vi "SSC DCPower Source Current v2.vi"(0 "DCPower SSC in":T1[](array[typedef]), 5 "Voltage Limit, V":dbl, 9 "Voltage Limit Range (V)":dbl format="%#_6p", 11 "error in":errorcluster, 12 "Current Level Range (A)":dbl=0.001 format="%#_13p", 14 "Current Level (A)":dbl format="%#_13g") -> (4 "DCPower SSC out":T1[](array[typedef]), 15 "error out":errorcluster)   [LabVIEW 2019]
uses:
  SSC DCPower.ctl
  <instrlib>/niDCPower/nidcpower.llb/niDCPower Output Function.ctl
  <instrlib>/niDCPower/nidcpower.llb/niDCPower Source Mode.ctl
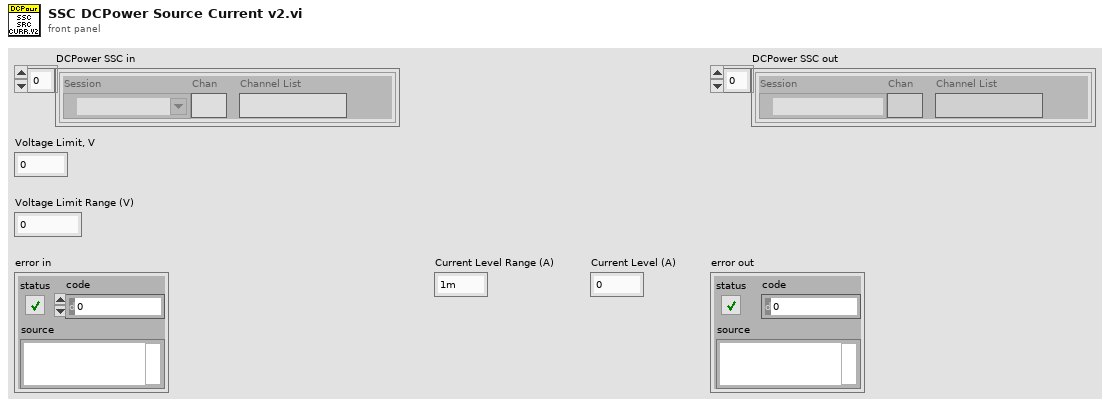
[diagram p1: front panel]
types:
  T1 = typedef "SSC DCPower.ctl" = cluster{"Session":refnum<k15>, "Chan":string, "Channel List":string}
  T2 = typedef "niDCPower Source Mode.ctl" = i32
  T3 = typedef "niDCPower Output Function.ctl" = i32
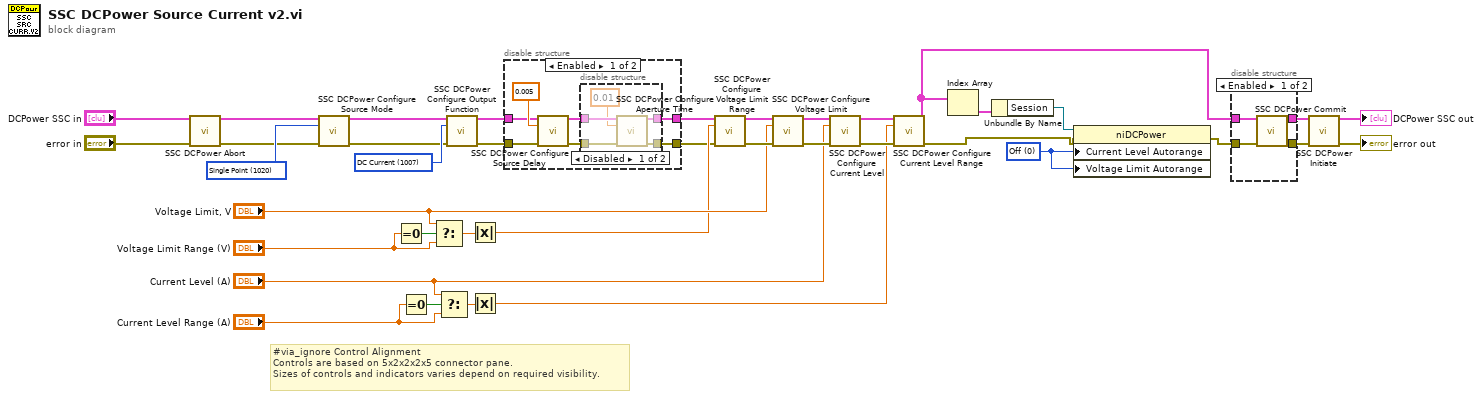
[diagram p0: block diagram]
diagram:
  w6 = 0 items=["Off", "On"] ("Source:DC Voltage:Voltage Level Autorange")
  w15 = T2 1020 items=["Single Point"=1020, "Sequence"=1021] ("Source Mode")
  w38 = T3 1007 items=["DC Voltage"=1006, "DC Current"=1007, "Pulse Voltage"=1049, "Pulse Current"=1050] ("Output Function")
  # "#via_ignore Control Alignment\nControls are based on 5x2x2x2x5 connector pane.\nSizes of controls and indicators varies depend on required visibility."
  n1 = call "SSC DCPower Abort.vi"("DCPower SSC in"="DCPower SSC in", "error in"="error in") -> ("DCPower SSC out"=w12:T1[], "error out"=w14:errorcluster)  [unwired: 12 in]
  n2 = call "SSC DCPower Configure Source Mode.vi"("DCPower SSC in"=w12, "Source Mode"=w15, "error in"=w14) -> ("DCPower SSC out"=w11:T1[], "error out"=w13:errorcluster)  [unwired: 11 in]
  n3 = Equal To 0?(x="Voltage Limit Range (V)") -> (x = 0?=w20:bool)
  n4 = Equal To 0?(x="Current Level Range (A)") -> (x = 0?=w25:bool)
  n5 = Select(t="Voltage Limit, V", s=w20, f="Voltage Limit Range (V)") -> (s? t:f=w17:dbl)
  n6 = Select(t="Current Level (A)", s=w25, f="Current Level Range (A)") -> (s? t:f=w22:dbl)
  n7 = call "SSC DCPower Configure Output Function.vi"("DCPower SSC in"=w11, "Output Function"=w38, "error in"=w13) -> ("DCPower SSC out"=w10:T1[], "error out"=w9:errorcluster)  [unwired: 11 in]
  n8 = Absolute Value(x=w17) -> (abs(x)=w16:dbl)
  n9 = Absolute Value(x=w22) -> (abs(x)=w21:dbl)
  n10 = disable-structure shown="Enabled" {
    disable-tunnel: w10 -> [w40 w54]
    disable-tunnel: [w44 w54] -> w8
    disable-tunnel: w9 -> [w39 w53]
    disable-tunnel: [w42 w53] -> w7
    frame Enabled {
      n11 = call "SSC DCPower Configure Source Delay.vi"("DCPower SSC in"=w40, "Source Delay (s)"=0.005, "error in"=w39) -> ("DCPower SSC out"=w45:T1[], "error out"=w43:errorcluster)  [unwired: 11 in]
      n12 = disable-structure shown="Disabled" {
        disable-tunnel: w45 -> [w50 w52]
        disable-tunnel: [w49 w52] -> w44
        disable-tunnel: w43 -> [w48 w51]
        disable-tunnel: [w47 w51] -> w42
        frame Disabled {
          n13 = call "SSC DCPower Configure Aperture Time.vi"("DCPower SSC in"=w50, "Aperture Time"=0.01, "error in"=w48) -> ("DCPower SSC out"=w49:T1[], "error out"=w47:errorcluster)  [unwired: 11 in]
        }
        frame Enabled {
        }
      }
    }
    frame Disabled {
    }
  }
  n14 = call "SSC DCPower Configure Voltage Limit Range.vi"("DCPower SSC in"=w8, "Voltage Limit Range (V)"=w16, "error in"=w7) -> ("DCPower SSC out"=w36:T1[], "error out"=w35:errorcluster)  [unwired: 11 in]
  n15 = call "SSC DCPower Configure Voltage Limit.vi"("DCPower SSC in"=w36, "Voltage Limit (V)"="Voltage Limit, V", "error in"=w35) -> ("DCPower SSC out"=w34:T1[], "error out"=w33:errorcluster)  [unwired: 11 in]
  n16 = call "SSC DCPower Configure Current Level.vi"("DCPower SSC in"=w34, "Current Level (A)"="Current Level (A)", "error in"=w33) -> ("DCPower SSC out"=w32:T1[], "error out"=w31:errorcluster)  [unwired: 11 in]
  n17 = call "SSC DCPower Configure Current Level Range.vi"("DCPower SSC in"=w32, "Current Level Range (A)"=w21, "error in"=w31) -> ("DCPower SSC out"=w3:T1[], "error out"=w2:errorcluster)  [unwired: 11 in]
  n18 = Index Array(array=w3) -> (element=w5:T1)  [unwired: 1 in]
  n19 = Unbundle By Name(w5) -> ("Session"=w4:refnum<k15>)
  n20 = property class="niDCPower"(reference=w4, error in=w2, "Current Level Autorange"=w6, "Voltage Limit Autorange"=w6) -> (error out=w1:errorcluster)  [unwired: 1 out]
  n21 = disable-structure shown="Enabled" {
    disable-tunnel: w1 -> [w55 w60]
    disable-tunnel: [w58 w60] -> w29
    disable-tunnel: w3 -> [w57 w59]
    disable-tunnel: [w56 w59] -> w27
    frame Enabled {
      n22 = call "SSC DCPower Commit.vi"("DCPower SSC in"=w57, "error in"=w55) -> ("DCPower SSC out"=w56:T1[], "error out"=w58:errorcluster)  [unwired: 12 in]
    }
    frame Disabled {
    }
  }
  n23 = call "SSC DCPower Initiate.vi"("DCPower SSC in"=w27, "error in"=w29) -> ("DCPower SSC out"=→"DCPower SSC out":T1[], "error out"=→"error out":errorcluster)  [unwired: 12 in]
